vi "Hopper_HW.vi"   [LabVIEW 2017]
uses:
  Globals/Global_STOP.vi
  Global_ShooterCTRL.vi
  <vilib>/Rock Robotics/WPI/ThirdParty/CanMotor/TalonSRX/WPI_CANTalonSRX_APIControlMode.ctl
types:
  T1 = typedef "WPI_CANTalonSRX_APIControlMode.ctl" = enum8{"Percent VBus", "Speed", "Position", "Slave", "Unchanged / Invalid", "Voltage Compensation", "Current", "Motion Profile", "Motion Magic"}
  T2 = typedef "WPI_MotorControlDeviceRef.ctl" = cluster{"DeviceStatus":errorcluster, "Type":T3, "PWM":cluster{"PWM Channel":T4, "DeadBand":T5}, "CAN":cluster{"Device Number":u8, "SetOutput VI Ref":variant, "GetOutput VI Ref":variant, "Enable VI Ref":variant, "Disable VI Ref":variant, "Data":variant}, "Invert":bool}
  T3 = typedef "WPI_MotorControlType.ctl" = enum16{"PWM", "CAN"}
  T4 = typedef "FPGA_DIOPWMChannel.ctl" = enum8{"PWM 0", "PWM 1", "PWM 2", "PWM 3", "PWM 4", "PWM 5", "PWM 6", "PWM 7", "PWM 8", "PWM 9", "PWM MXP 0", "PWM MXP 1", "PWM MXP 2", "PWM MXP 3", "PWM MXP 4", "PWM MXP 5", "PWM MXP 6", "PWM MXP 7", "PWM MXP 8", "PWM MXP 9", "Invalid"}
  T5 = typedef "WPI_PWMDeadband.ctl" = cluster{"Name":string, "maxPositivePwm":i32, "minPositivePwm":i32, "centerPwm":i32, "maxNegativePwm":i32, "minNegativePwm":i32, "angularRange":u16}
  T6 = typedef "WPI_MotorControlDeviceRef.ctl" = cluster{"DeviceStatus":errorcluster, "Type":T7, "PWM":cluster{"PWM Channel":T4, "DeadBand":T5}, "CAN":cluster{"Device Number":u8, "SetOutput VI Ref":variant, "GetOutput VI Ref":variant, "Enable VI Ref":variant, "Disable VI Ref":variant, "Data":variant}, "Invert":bool, "DIO PWM":cluster{"PWM \"Enable\" Channel":T4, "DIOChannel":T8, "PWM Rate":dbl}}
  T7 = typedef "WPI_MotorControlType.ctl" = enum16{"PWM", "CAN", "DIO PWM"}
  T8 = typedef "FPGA_DIOChannel.ctl" = enum8{"DIO 0", "DIO 1", "DIO 2", "DIO 3", "DIO 4", "DIO 5", "DIO 6", "DIO 7", "DIO 8", "DIO 9", "DIO MXP 0", "DIO MXP 1", "DIO MXP 2", "DIO MXP 3", "DIO MXP 4", "DIO MXP 5", "DIO MXP 6", "DIO MXP 7", "DIO MXP 8", "DIO MXP 9", "DIO MXP 10", "DIO MXP 11", "DIO MXP 12", "DIO MXP 13", "DIO MXP 14", "DIO MXP 15", "SPI Port CS1", "SPI Port CS2", "SPI Port CS3", "SPI Port MISO", "SPI Port MOSI", "Invalid"}
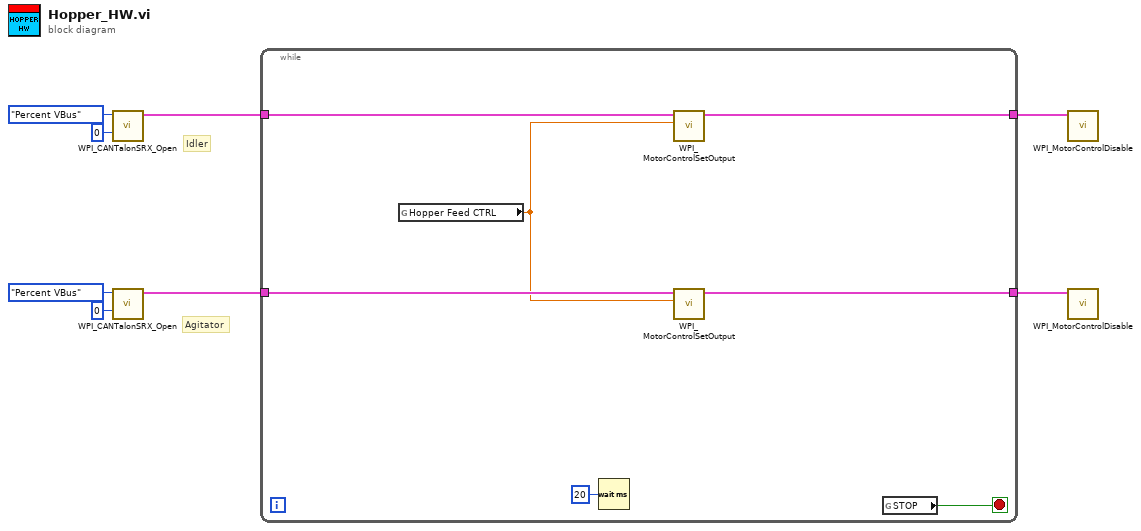
[diagram p0: block diagram]
diagram:
  # "Agitator"
  # "Idler"
  n1 = call <vilib>:"WPI_CANTalonSRX_Open.vi"("Device Number"=u8 0, "Control Mode"=WPI_CANTalonSRX_APIControlMode."Percent VBus") -> ("CAN Talon SRX Ref"=w1:T2)  [unwired: 8 in, 1 out]
  n2 = call <vilib>:"WPI_CANTalonSRX_Open.vi"("Device Number"=u8 0, "Control Mode"=WPI_CANTalonSRX_APIControlMode."Percent VBus") -> ("CAN Talon SRX Ref"=w3:T2)  [unwired: 8 in, 1 out]
  n3 = while {
    tunnel: w1 -> [w13]
    tunnel: [w12] -> w2
    tunnel: w3 -> [w11]
    tunnel: [w10] -> w4
    stop <- w15 stop-if-true
    n4 = global read "Global_ShooterCTRL.vi" "Hopper Feed CTRL"() -> (w9:dbl)
    n5 = Wait (ms)(milliseconds to wait=u32 20) -> ()  [unwired: 1 out]
    n6 = call <vilib>:"WPI_MotorControlSetOutput.vi"("Output"=w9, "MotorControlDevRef"=w13) -> ("MotorControlDevRef"=w12:T6)  [unwired: 7 in, 2 out]
    n7 = call <vilib>:"WPI_MotorControlSetOutput.vi"("Output"=w9, "MotorControlDevRef"=w11) -> ("MotorControlDevRef"=w10:T6)  [unwired: 7 in, 2 out]
    n8 = global read "Global_Stop.vi" "STOP"() -> (w15:bool)
  }
  n9 = call <vilib>:"WPI_MotorControlDisable.vi"("MotorControlDevRef"=w2) -> ()  [unwired: 9 in, 2 out]
  n10 = call <vilib>:"WPI_MotorControlDisable.vi"("MotorControlDevRef"=w4) -> ()  [unwired: 9 in, 2 out]
